vi "Convert AI with Conversion Time Module to Slot Configuration.vi"(8 "error in":errorcluster, 9 "module in":refnum<class "Module.lvclass">, 10 "9224 in":refnum<class "9224.lvclass">, 11 "slot ref in":T1 format="%.0x") -> (0 "error out":errorcluster, 3 "slot ref out":T1 format="%.0x")   [LabVIEW 2017, in "Scan Engine Scripting.lvlib"]
uses:
  Scan Engine Scripting.lvlib
  <vilib>/NI Veristand/Custom Device API/Custom Device Item Ref.ctl
  Modules/Module/Module.lvclass
  Modules.lvlibp/9224/9224.lvclass
  C:/Users/nitest/Documents/niveristand-scan-engine-ethercat-custom-device/Custom Device Source/Modules.lvlibp/RSI Module/RSI Module.lvclass
  Modules.lvlibp/RSI Module/RSI Module.lvclass
  <vilib>/NI Veristand/Custom Device API/Custom Device API.lvlib
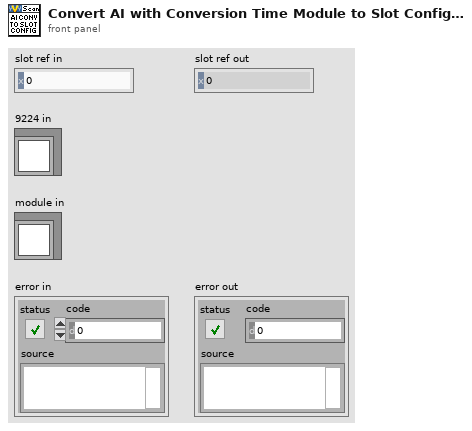
[diagram p1: front panel]
types:
  T1 = typedef "Custom Device API.lvlib/Custom Device Item Ref.ctl" = u64
  T2 = typedef "Scan Engine Scripting.lvlib/analog channel settings.ctl" = cluster{"name":string, "default value":dbl}
  T3 = typedef "Scan Engine Scripting.lvlib/Analog Input with Conversion Time Mode.lvclass/Conversion Time.ctl" = enum16{"High Speed (1k S/s)", "Medium Speed (100 S/s)", "Medium Resolution (50/60Hz Rejection - 12 S/s)", "High Resolution (50/60Hz Rejection - 2 S/s)"}
  T4 = typedef "Modules.lvlibp/Custom Device API.lvlib/Custom Device Item Ref.ctl" = u64
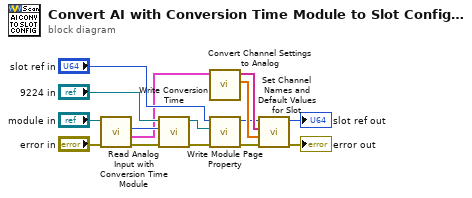
[diagram p0: block diagram]
diagram:
  n1 = call-dynamic "Read Analog Input with Conversion Time Module.vi"("error in"="error in", "module in"="module in") -> ("error out"=w3:errorcluster, "channel settings"=w4:T2[], "conversion time"=w5:T3)  [unwired: 6 in, 1 out]
  n2 = call-dynamic "Write Conversion Time.vi"("error in"=w3, "Conversion Time"=w5, "9224 in"="9224 in") -> ("error out"=w2:errorcluster, "9224 out"=w8:refnum<class "9224.lvclass">)  [unwired: 7 in]
  n3 = call "Convert Channel Settings to Analog.vi"("channel settings"=w4) -> ("channel default values"=w15:dbl[], "channel names"=w14:string[])  [unwired: 9 in]
  n4 = call "Write Module Page Property.vi"("error in (no error)"=w2, "RSI Module"=w8, "Node Ptr In"="slot ref in") -> ("error out"=w1:errorcluster, "Node Ptr Out"=w6:T4)  [unwired: 6 in, 1 out]
  n5 = call "Set Channel Names and Default Values for Slot.vi"("error in"=w1, "default values"=w15, "channel names"=w14, "slot ref in"=w6) -> ("error out"=→"error out":errorcluster, "slot ref out"=→"slot ref out":T1)  [unwired: 6 in]
